vi "Coherent global.vi"() -> ()   [LabVIEW 2014]
panel:
  out "DLL path":path
  out "Blue laser hDev index":i32=-1
  out "Green laser hDev index":i32=-1
  in  "Blue laser serial no.":string
  in  "Green laser serial no.":string
  out "Device handles":u32[](array[numeric])
  out "Number of connected devices":u32
  # "PN 06/11/2014"
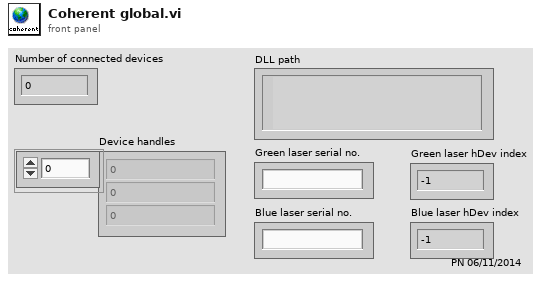
[diagram p1: front panel]
diagram:
